vi "do_waveform_pc_infinite.vi"() -> ()   [LabVIEW 2020]
uses:
  <vilib>/Waveform/DWDTOps.llb/DWDT Analog to Digital.vi
panel:
  out "x-y":u32
  out "Rounds":i32
  in  "Stop":bool
  out "数字波形图":digitalwaveform(graph)={"t0"=timestamp(0 s since 1904-01-01), "dt"=1e-05, "Y"={"transitions"=[0, 1, 2, 3, 4, 5], "data"=[[0, 0, 0, 0], [0, 1, 0, 1], [1, 0, 1, 0], [0, 0, 0, 1], [1, 0, 0, 1], [0, 0, 0, 0]]}}
  out "error out":errorcluster caption="错误输出"
  in  "SamplePeriod(ns)":u32=10000
  in  "DevIndex":i32
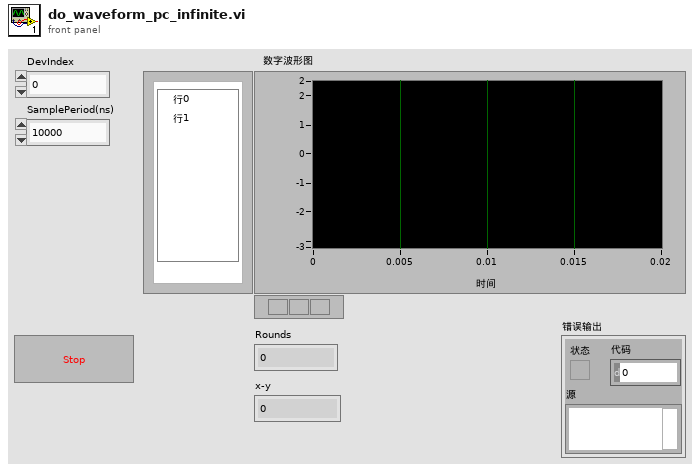
[diagram p1: front panel]
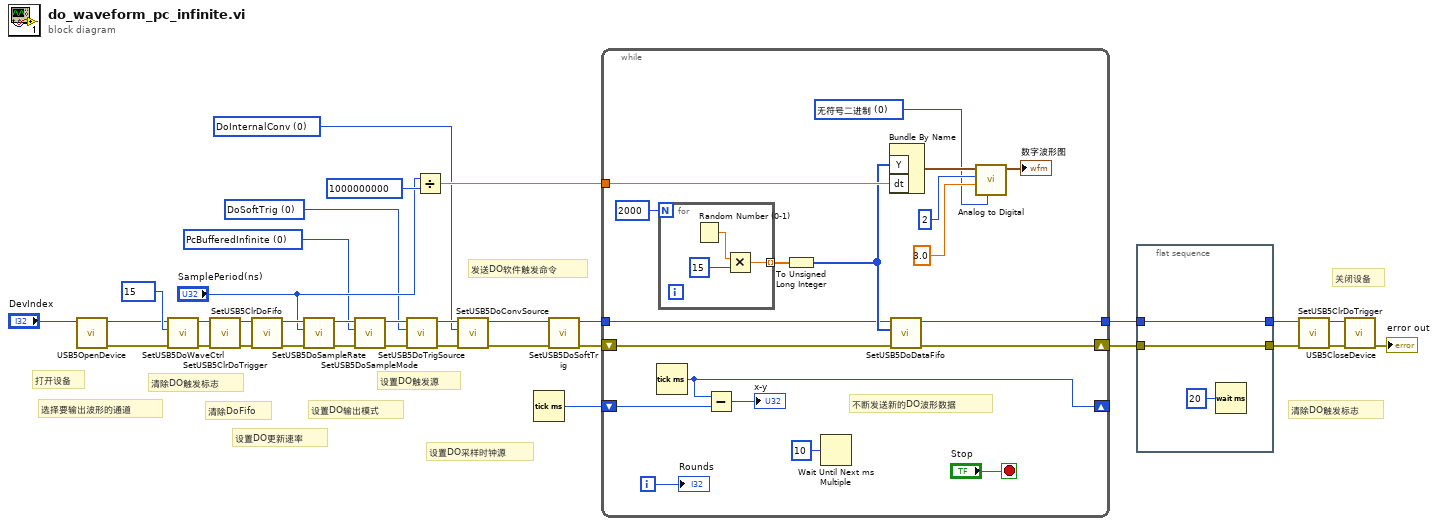
[diagram p0: block diagram]
diagram:
  w1 = u8 0 items=["DoInternalConv"=0, "ConvIn"=1, "AiConv"=2, "DiConv"=3, "Ao0Conv"=5, "Ao1Conv"=6, "Ao2Conv"=7, "Ao3Conv"=8] ("DoConvSource")
  w2 = u8 0 items=["DoSoftTrig"=0, "ExtTrigIn"=1, "Din0RisingEdge"=2, "Din1RisingEdge"=3, "Din2RisingEdge"=4, "Din3RisingEdge"=5, "WithAiTrig"=6, "WithDiTrig"=7, "WithAo0Trig"=9, "WithAo1Trig"=10, "WithAo2Trig"=11, "WithAo3Trig"=12, "GlobalSoftTrig"=255] ("DoTrigSource")
  w3 = u8 0 items=["PcBufferedInfinite", "NCycle"] ("DoSampleMode")
  # "关闭设备"
  # "清除DO触发标志"
  # "发送DO软件触发命令"
  # "设置DO采样时钟源"
  # "设置DO触发源"
  # "设置DO输出模式"
  # "设置DO更新速率"
  # "清除DoFifo"
  # "清除DO触发标志"
  # "选择要输出波形的通道"
  # "打开设备"
  n1 = call "USB5OpenDevice.vi"("DevIndex"="DevIndex") -> ("error out"=w5:errorcluster, "DevIndex Out"=w6:i32)  [unwired: 9 in]
  n2 = call "SetUSB5DoWaveCtrl.vi"("错误输入（无错误）"=w5, "Chan"=u32 15, "DevIndex"=w6) -> ("错误输出"=w25:errorcluster, "DevIndex Out"=w26:i32)  [unwired: 7 in]
  n3 = call "SetUSB5ClrDoTrigger.vi"("错误输入（无错误）"=w25, "DevIndex"=w26) -> ("错误输出"=w31:errorcluster, "DevIndex Out"=w32:i32)  [unwired: 8 in]
  n4 = call "SetUSB5ClrDoFifo.vi"("错误输入（无错误）"=w31, "DevIndex"=w32) -> ("错误输出"=w29:errorcluster, "DevIndex Out"=w30:i32)  [unwired: 8 in]
  n5 = call "SetUSB5DoSampleRate.vi"("错误输入（无错误）"=w29, "SamplePeriod(ns)"="SamplePeriod(ns)", "DevIndex"=w30) -> ("错误输出"=w22:errorcluster, "DevIndex Out"=w23:i32)  [unwired: 7 in]
  n6 = call "SetUSB5DoSampleMode.vi"("错误输入（无错误）"=w22, "DoSampleMode"=w3, "DevIndex"=w23) -> ("错误输出"=w20:errorcluster, "DevIndex Out"=w21:i32)  [unwired: 7 in]
  n7 = call "SetUSB5DoTrigSource.vi"("错误输入（无错误）"=w20, "DoTrigSource"=w2, "DevIndex"=w21) -> ("错误输出"=w18:errorcluster, "DevIndex Out"=w19:i32)  [unwired: 7 in]
  n8 = Divide(x="SamplePeriod(ns)", y=u32 1000000000) -> (x/y=w27:dbl)
  n9 = call "SetUSB5DoConvSource.vi"("错误输入（无错误）"=w18, "DoConvSource"=w1, "DevIndex"=w19) -> ("错误输出"=w16:errorcluster, "DevIndex Out"=w17:i32)  [unwired: 7 in]
  n10 = Tick Count (ms)() -> (millisecond timer value=w7:u32)
  n11 = call "SetUSB5DoSoftTrig.vi"("错误输入（无错误）"=w16, "DevIndex"=w17) -> ("错误输出"=w13:errorcluster, "DevIndex Out"=w15:i32)  [unwired: 8 in]
  n12 = while {
    tunnel: w27 -> [w48]
    tunnel: w15 -> [w43]
    tunnel: [w42] -> w14
    shift-right: [w40] -> w12
    shift-left: w13 -> [w41]
    shift-right: [w35] -> _
    shift-left: w7 -> [w37]
    i -> [w38]
    stop <- "Stop" stop-if-true
    w50 = u16 0 items=["无符号二进制", "二进制偏移量", "二进制补码"] ("data format (offset binary)")
    # "不断发送新的DO波形数据"
    n13 = Tick Count (ms)() -> (millisecond timer value=w35:u32)
    n14 = for {
      N: 2000 -> [_]
      tunnel: [w54] -> w45 mode=indexing
      n15 = Random Number (0-1)() -> (number: 0 to 1=w55:dbl)
      n16 = Multiply(x=w55, y=15) -> (x*y=w54:dbl)
    }
    n17 = Subtract(x=w35, y=w37) -> (x-y=→"x-y":u32)
    n18 = To Unsigned Long Integer(number=w45) -> (unsigned 32bit integer=w44:u32[])
    n19 = Wait Until Next ms Multiple(millisecond multiple=u32 10 ("毫秒倍数")) -> ()  [unwired: 1 out]
    n20 = Bundle By Name ("创建波形")("Y"=w44, "dt"=w48) -> (w53:waveform(u32))  [unwired: 1 in]
    n21 = call "SetUSB5DoDataFifo.vi"("错误输入（无错误）"=w41, "Value"=w44, "DevIndex"=w43) -> ("错误输出"=w40:errorcluster, "DevIndex Out"=w42:i32)  [unwired: 7 in]
    n22 = call-poly <vilib>:"Analog to Digital.vi"("data format (offset binary)"=w50, "full-scale range (pk-pk)"=3.0, "resolution (16 bit)"=2, "analog waveform"=w53) -> ("digital waveform"=→"数字波形图":digitalwaveform)  [unwired: 4 in, 3 out]
    "Rounds" <- w38
  }
  n23 = flat-sequence {
    tunnel: [w59] -> w10
    tunnel: w14 -> [w59]
    tunnel: [w58] -> w11
    tunnel: w12 -> [w58]
    frame #0 {
      n24 = Wait (ms)(milliseconds to wait=u32 20 ("等待时间（毫秒）")) -> ()  [unwired: 1 out]
    }
  }
  n25 = call "SetUSB5ClrDoTrigger.vi"("错误输入（无错误）"=w11, "DevIndex"=w10) -> ("错误输出"=w8:errorcluster, "DevIndex Out"=w9:i32)  [unwired: 8 in]
  n26 = call "USB5CloseDevice.vi"("错误输入（无错误）"=w8, "DevIndex"=w9) -> ("error out"=→"error out":errorcluster)  [unwired: 8 in, 1 out]
